vi "Parse Status Channels.vi"(5 "FIFO Idx Qs":T2, 8 "error in":errorcluster, 11 "Device Reference in":T1 format="%.0x") -> (0 "error out":errorcluster, 2 "Status Config":T3 {"HWOut Dur Ref" format="%.0x"; "HWIn Dur Ref" format="%.0x"; "HWOut Count Ref" format="%.0x"; "HWIn Count Ref" format="%.0x"; "Error Data Ref" format="%.0x"}, 3 "Device Ref out":T1 format="%.0x")   [LabVIEW 2011, in "AIT 1553 Custom Device.lvlib"]
uses:
  AIT 1553 Custom Device.lvlib
  RT Controls/Status Channels Config.ctl
  <vilib>/NI Veristand/Custom Device API/Data Reference.ctl
  RT Controls/FIFO Idx Qs.ctl
  <vilib>/NI Veristand/Custom Device API/Custom Device Item Ref.ctl
  <vilib>/NI Veristand/Custom Device API/Data Access Type.ctl
  RT Controls/Data Ref FGV Command.ctl
  <vilib>/NI Veristand/Custom Device Tools/Custom Device Utility Library/NI VeriStand - Search for Item by Name.vi
  Controls and Global/Global.vi
  <vilib>/NI Veristand/Custom Device Tools/Custom Device Utility Library/Custom Device Utility Library.lvlib
  <vilib>/NI Veristand/Custom Device API/Custom Device API.lvlib
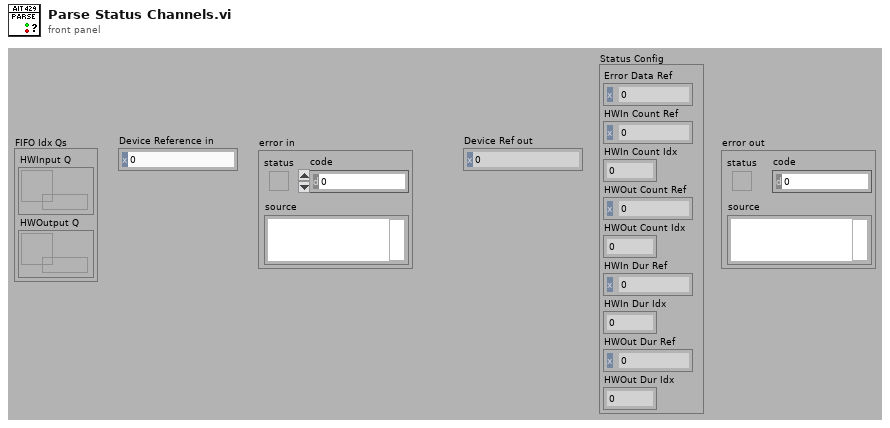
[diagram p1: front panel]
types:
  T1 = typedef "Custom Device API.lvlib/Custom Device Item Ref.ctl" = u64
  T2 = typedef "AIT 1553 Custom Device.lvlib/FIFO Idx Qs.ctl" = cluster{"HWInput Q":refnum<queue>, "HWOutput Q":refnum<queue>}
  T3 = typedef "AIT 1553 Custom Device.lvlib/Status Channels Config.ctl" = cluster{"Error Data Ref":T4, "HWIn Count Ref":T4, "HWIn Count Idx":i32, "HWOut Count Ref":T4, "HWOut Count Idx":i32, "HWIn Dur Ref":T4, "HWIn Dur Idx":i32, "HWOut Dur Ref":T4, "HWOut Dur Idx":i32}
  T4 = typedef "Custom Device API.lvlib/Data Reference.ctl" = i32
  T5 = typedef "AIT 1553 Custom Device.lvlib/Data Ref FGV Command.ctl" = enum16{"Intialize", "Get", "Update"}
  T6 = typedef "Custom Device API.lvlib/Data Access Type.ctl" = enum16{"Read", "Write"}
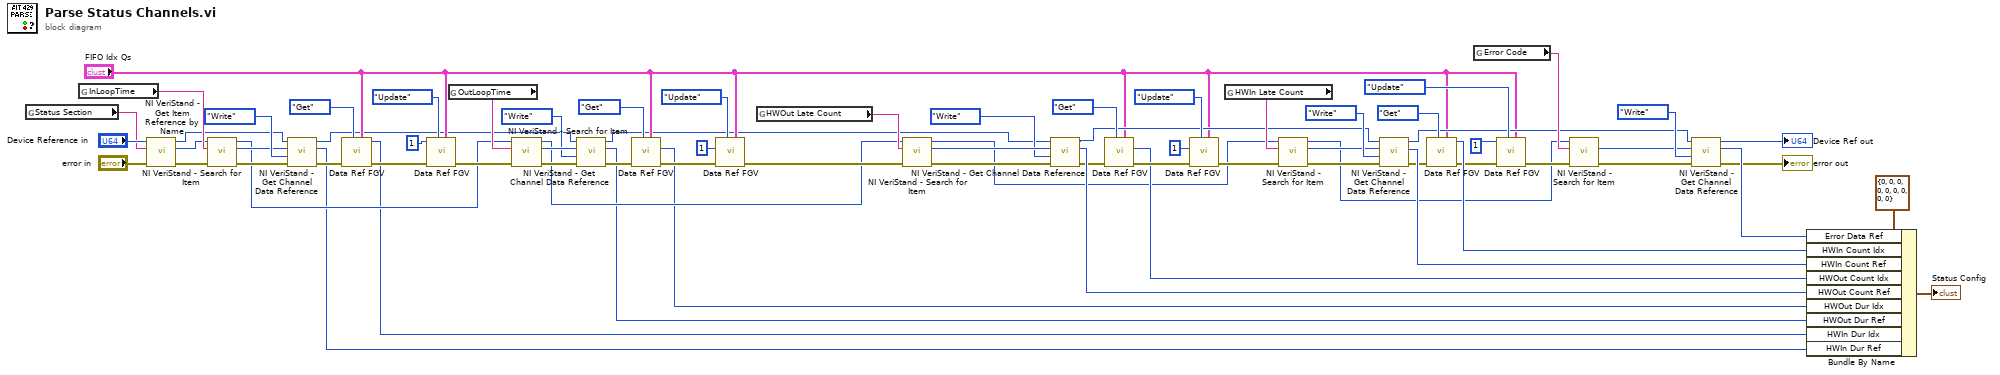
[diagram p0: block diagram]
diagram:
  n1 = global read "Global.vi" "Status Section"() -> (w38:string)
  n2 = global read "Global.vi" "InLoopTime"() -> (w32:string)
  n3 = call <vilib>:"NI VeriStand - Get Item Reference by Name.vi"("error in (no error)"="error in", "Item Name"=w38, "Parent Ref in"="Device Reference in") -> ("error out"=w14:errorcluster, "Item Ref"=w15:T1, "Parent Ref out"=w13:T1)  [unwired: 5 in, 1 out]
  n4 = call-poly <vilib>:"NI VeriStand - Search for Item.vi"("error in"=w14, "Item Name"=w32, "Section Ref in"=w15) -> ("error out"=w30:errorcluster, "Item Ref"=w29:T1, "Section Ref out"=w9:T1)  [unwired: 5 in, 1 out]
  n5 = call <vilib>:"NI VeriStand - Get Channel Data Reference.vi"("error in (no error)"=w30, "Access"=Data_Access_Type."Write", "Channel Ref in"=w29, "Device Ref in"=w13) -> ("error out"=w28:errorcluster, "Channel Data Reference"=w1:T4, "Device Ref out"=w5:T1)  [unwired: 5 in]
  n6 = call "Data Ref FGV.vi"("FIFO Idx Qs"="FIFO Idx Qs", "Command"=Data_Ref_FGV_Command."Get", "error in (no error)"=w28) -> ("error out"=w26:errorcluster, "HWInput FIFO Index / Length"=w2:i32)  [unwired: 6 in, 1 out]
  n7 = call "Data Ref FGV.vi"("FIFO Idx Qs"="FIFO Idx Qs", "Command"=Data_Ref_FGV_Command."Update", "error in (no error)"=w26, "HWInput Length"=1) -> ("error out"=w12:errorcluster)  [unwired: 5 in, 2 out]
  n8 = global read "Global.vi" "OutLoopTime"() -> (w17:string)
  n9 = call-poly <vilib>:"NI VeriStand - Search for Item.vi"("error in"=w12, "Item Name"=w17, "Section Ref in"=w9) -> ("error out"=w19:errorcluster, "Item Ref"=w20:T1, "Section Ref out"=w8:T1)  [unwired: 5 in, 1 out]
  n10 = call <vilib>:"NI VeriStand - Get Channel Data Reference.vi"("error in (no error)"=w19, "Access"=Data_Access_Type."Write", "Channel Ref in"=w20, "Device Ref in"=w5) -> ("error out"=w21:errorcluster, "Channel Data Reference"=w3:T4, "Device Ref out"=w4:T1)  [unwired: 5 in]
  n11 = call "Data Ref FGV.vi"("FIFO Idx Qs"="FIFO Idx Qs", "Command"=Data_Ref_FGV_Command."Get", "error in (no error)"=w21) -> ("error out"=w23:errorcluster, "HWOutput FIFO Index / Length"=w6:i32)  [unwired: 6 in, 1 out]
  n12 = call "Data Ref FGV.vi"("FIFO Idx Qs"="FIFO Idx Qs", "Command"=Data_Ref_FGV_Command."Update", "error in (no error)"=w23, "HWOutput Length"=1 ("HWInput Length")) -> ("error out"=w11:errorcluster)  [unwired: 5 in, 2 out]
  n13 = global read "Global.vi" "HWOut Late Count"() -> (w48:string)
  n14 = call-poly <vilib>:"NI VeriStand - Search for Item.vi"("error in"=w11, "Item Name"=w48, "Section Ref in"=w8) -> ("error out"=w50:errorcluster, "Item Ref"=w51:T1, "Section Ref out"=w35:T1)  [unwired: 5 in, 1 out]
  n15 = call <vilib>:"NI VeriStand - Get Channel Data Reference.vi"("error in (no error)"=w50, "Access"=Data_Access_Type."Write", "Channel Ref in"=w51, "Device Ref in"=w4) -> ("error out"=w58:errorcluster, "Channel Data Reference"=w61:T4, "Device Ref out"=w36:T1)  [unwired: 5 in]
  n16 = call "Data Ref FGV.vi"("FIFO Idx Qs"="FIFO Idx Qs", "Command"=Data_Ref_FGV_Command."Get", "error in (no error)"=w58) -> ("error out"=w62:errorcluster, "HWOutput FIFO Index / Length"=w42:i32)  [unwired: 6 in, 1 out]
  n17 = call "Data Ref FGV.vi"("FIFO Idx Qs"="FIFO Idx Qs", "Command"=Data_Ref_FGV_Command."Update", "error in (no error)"=w62, "HWOutput Length"=1 ("HWInput Length")) -> ("error out"=w64:errorcluster)  [unwired: 5 in, 2 out]
  n18 = global read "Global.vi" "HWIn Late Count"() -> (w55:string)
  n19 = call-poly <vilib>:"NI VeriStand - Search for Item.vi"("error in"=w64, "Item Name"=w55, "Section Ref in"=w35) -> ("error out"=w53:errorcluster, "Item Ref"=w52:T1, "Section Ref out"=w33:T1)  [unwired: 5 in, 1 out]
  n20 = call <vilib>:"NI VeriStand - Get Channel Data Reference.vi"("error in (no error)"=w53, "Access"=Data_Access_Type."Write", "Channel Ref in"=w52, "Device Ref in"=w36) -> ("error out"=w56:errorcluster, "Channel Data Reference"=w68:T4, "Device Ref out"=w34:T1)  [unwired: 5 in]
  n21 = call "Data Ref FGV.vi"("FIFO Idx Qs"="FIFO Idx Qs", "Command"=Data_Ref_FGV_Command."Get", "error in (no error)"=w56) -> ("error out"=w65:errorcluster, "HWInput FIFO Index / Length"=w69:i32)  [unwired: 6 in, 1 out]
  n22 = global read "Global.vi" "Error Code"() -> (w37:string)
  n23 = call "Data Ref FGV.vi"("FIFO Idx Qs"="FIFO Idx Qs", "Command"=Data_Ref_FGV_Command."Update", "error in (no error)"=w65, "HWInput Length"=1) -> ("error out"=w66:errorcluster)  [unwired: 5 in, 2 out]
  n24 = call-poly <vilib>:"NI VeriStand - Search for Item.vi"("error in"=w66, "Item Name"=w37, "Section Ref in"=w33) -> ("error out"=w43:errorcluster, "Item Ref"=w46:T1)  [unwired: 5 in, 2 out]
  n25 = call <vilib>:"NI VeriStand - Get Channel Data Reference.vi"("error in (no error)"=w43, "Access"=Data_Access_Type."Write", "Channel Ref in"=w46, "Device Ref in"=w34) -> ("error out"=→"error out":errorcluster, "Channel Data Reference"=w67:T4, "Device Ref out"=→"Device Ref out":T1)  [unwired: 5 in]
  n26 = Bundle By Name(cluster=T3 {"Error Data Ref"=0, "HWIn Count Ref"=0, "HWIn Count Idx"=0, "HWOut Count Ref"=0, "HWOut Count Idx"=0, "HWIn Dur Ref"=0, "HWIn Dur Idx"=0, "HWOut Dur Ref"=0, "HWOut Dur Idx"=0} ("Stat Chn Cfg"), "Error Data Ref"=w67, "HWIn Count Idx"=w69, "HWIn Count Ref"=w68, "HWOut Count Idx"=w42, "HWOut Count Ref"=w61, "HWOut Dur Idx"=w6, "HWOut Dur Ref"=w3, "HWIn Dur Idx"=w2, "HWIn Dur Ref"=w1) -> (→"Status Config":T3)
